vi "Instrument-Template.doSomethingExample.vi"(8 "error in (no error)":errorcluster, 10 "Data":variant, 11 "Instrument.Transport in":refnum<class "Inst.Transport.lvclass">) -> (0 "error out":errorcluster, 2 "Data out":variant, 3 "Instrument.Transport out":refnum<class "Inst.Transport.lvclass">)   [LabVIEW 2019]
uses:
  Inst.Transport.lvclass
  Inst.Transport.lvclass/Inst.Transport.ctl
  <userlib>/LevyLab/Instrument Framework/subsystems/HAL/HAL.lvclass
  C:/Program Files (x86)/National Instruments/LabVIEW 2019/user.lib/LevyLab/Instrument Framework/Instrument Types/SCPI/Instrument.SCPI.lvclass
  C:/Program Files (x86)/National Instruments/LabVIEW 2019/user.lib/LevyLab/Instrument Framework/Instrument/Instrument.lvclass
  C:/Program Files (x86)/National Instruments/LabVIEW 2019/vi.lib/JKI/JKI SMO/SMO/SMO.lvclass
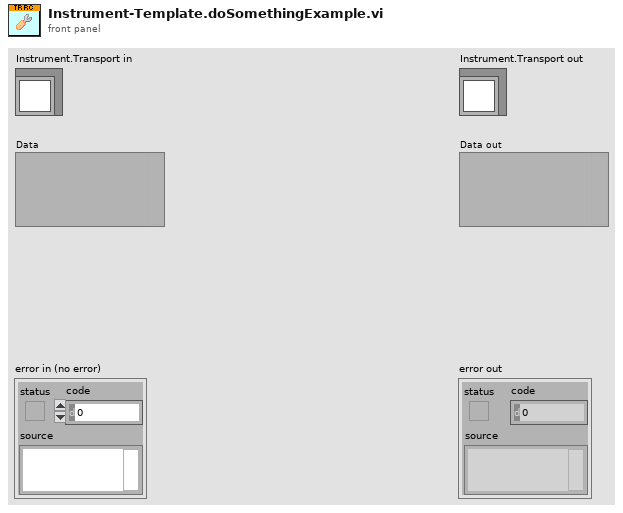
[diagram p1: front panel]
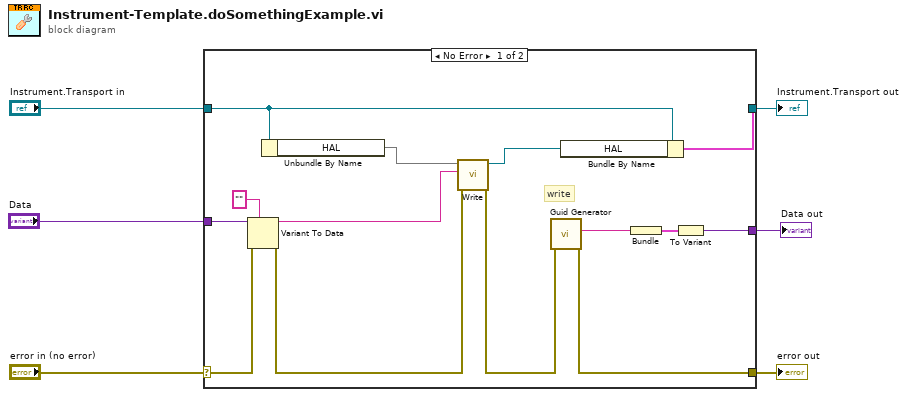
[diagram p0: block diagram]
diagram:
  n1 = case shown="No Error" "error in (no error)" {
    selector: "error in (no error)" -> [w18 w22]
    tunnel: [w16 w22] -> w5
    tunnel: [w7 w21] -> w3
    tunnel: "Instrument.Transport in" -> [w8 w21]
    tunnel: "Data" -> [w20 _]
    tunnel: [w15 _] -> w1
    frame No Error {
      # "write"
      n2 = Variant To Data(error in=w18, type="", Variant=w20) -> (data=w12:string, error out=w11:errorcluster)
      n3 = Unbundle By Name(w8) -> ("HAL"=w10)
      n4 = call-dynamic "Write.vi"("error in (no error)"=w11, "command"=w12, "HAL in"=w10) -> ("error out"=w13:errorcluster, "HAL out"=w9:refnum<class "HAL.lvclass">)  [unwired: 7 in]
      n5 = call <vilib>:"Guid Generator.vi"("error in (no error)"=w13) -> ("error out"=w16:errorcluster, "GUID"=w17:string)  [unwired: 9 in]
      n6 = Bundle By Name(cluster=w8, "HAL"=w9) -> (w7:cluster{})
      n7 = Bundle("GUID"=w17) -> (w14:cluster{"GUID":string})  [unwired: 1 in]
      n8 = To Variant(anything=w14) -> (Variant=w15:variant)
    }
    frame Error {
    }
  }
  "error out" <- w5
  "Instrument.Transport out" <- w3
  "Data out" <- w1
